vi "SaveConfig.vi"(8 "error in (no error)":errorcluster, 11 "Config":T1={"Path"="C:\\Glass", "Days to Keep"=30, "Number of Rows"=90}) -> (0 "error out":errorcluster)   [LabVIEW 2015, in "ConfigHelper.lvlib"]
uses:
  ConfigHelper.lvlib
  Config.ctl
  <vilib>/addons/PointValueMap/subVIs/Point_Write_variant.vi
  <vilib>/addons/PointValueMap/PointValueMap.lvlib
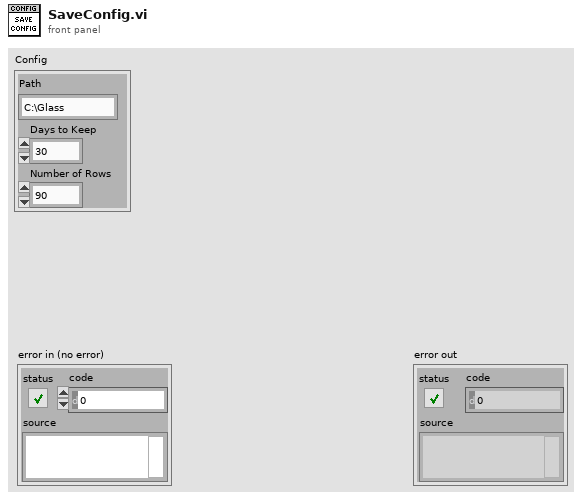
[diagram p1: front panel]
types:
  T1 = typedef "ConfigHelper.lvlib/Config.ctl" = cluster{"Path":string, "Days to Keep":i32, "Number of Rows":i32}
  T2 = typedef "PointValueMap.lvlib/PointMap.ctl" = refnum<data-value>
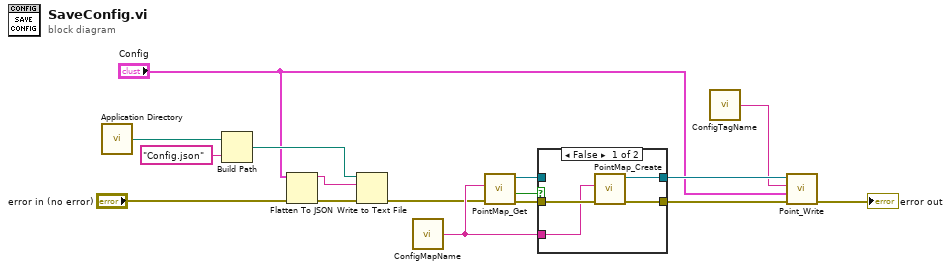
[diagram p0: block diagram]
diagram:
  n1 = call <vilib>:"Application Directory.vi"() -> ("Application Directory"=w16:path)
  n2 = Build Path(base path=w16, name or relative path="Config.json") -> (appended path=w14:path)
  n3 = Flatten To JSON(anything="Config", error in (no error)="error in (no error)") -> (JSON string=w11:string, 11:w12:errorcluster)  [unwired: 1 in]
  n4 = Write to Text File(file (use dialog)=w14, text=w11, error in=w12) -> (error out=w2:errorcluster)  [unwired: 1 in, 2 out]
  n5 = call "ConfigMapName.vi"() -> ("Name"=w5:string)  [unwired: 5 in]
  n6 = call <vilib>:"PointMap_Get.vi"("error in (no error)"=w2, "Name"=w5) -> ("error out"=w9:errorcluster, "Found?"=w10:bool, "Map Out"=w8:T2)  [unwired: 7 in]
  n7 = case shown="False" w10 {
    tunnel: w9 -> [w20 w21]
    tunnel: w8 -> [_ w22]
    tunnel: w5 -> [w19 _]
    tunnel: [w18 w22] -> w6
    tunnel: [w17 w21] -> w7
    frame False {
      n8 = call <vilib>:"PointMap_Create.vi"("error in (no error)"=w20, "Name"=w19) -> ("error out"=w17:errorcluster, "Map Out"=w18:T2)  [unwired: 8 in]
    }
    frame True {
    }
  }
  n9 = call "ConfigTagName.vi"() -> ("Name"=w4:string)  [unwired: 5 in]
  n10 = call-poly <vilib>:"Point_Write.vi"("Error In"=w7, "Value"="Config", "Tag"=w4, "Map"=w6) -> ("Error Out"=→"error out":errorcluster)  [unwired: 6 in, 1 out]
